vi "ScriptHelper.vi"(11 "Tag":string) -> ()   [LabVIEW 2018]
uses:
  AvailableModules.ctl
  NistPluggableModules/TestClass/Test.lvclass
  NistPluggableModules/Visualization/VisualizeBase/VisualizeBase_class/VisualizeBase.lvclass
panel:
  in  "Select Module":T1
  in  "Available Commands":i32(listbox)
  out "Command Information":string
  # "*Drag and drop Available Commands or selectedexample commands into the script editor"
  # "Available Commands"
  # "Command Information"
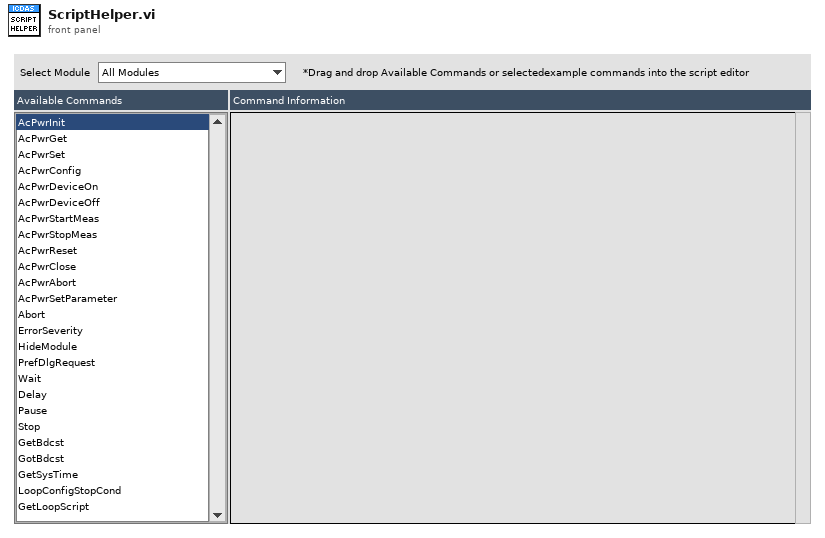
[diagram p1: front panel]
types:
  T1 = typedef "AvailableModules.ctl" = enum16{"All Modules", "AcPwr", "Analysis", "Digitizer", "FGen", "Scope", "Sensor", "Sync"}
  T2 = typedef "Plugin Tree Tag.ctl" = cluster{"ItemType":T3, "Name":string, "Path":path, "Script":string[]}
  T3 = typedef "Plugins Tree Item Type.ctl" = enum16{"Plugin", "Instrument", "INI File", "INI Script"}
  T4 = typedef "Test.lvclass/INIInfo.ctl" = cluster{"Module Name":string, "INI File Name":string, "Class Name":string, "INI File Name Without Extension":string, "Module.Class.INI File Name":string, "Visualization VI Path":path, "Instrument Class Path":path}
  T5 = typedef "Visualization.lvlib/VisualizeBase.lvclass/VisFrmWrkBroadcastEvents.ctl" = cluster{"StatusUpdate":refnum<user-event>, "DidStop":refnum<user-event>, "NewModuleLoaded":refnum<user-event>}
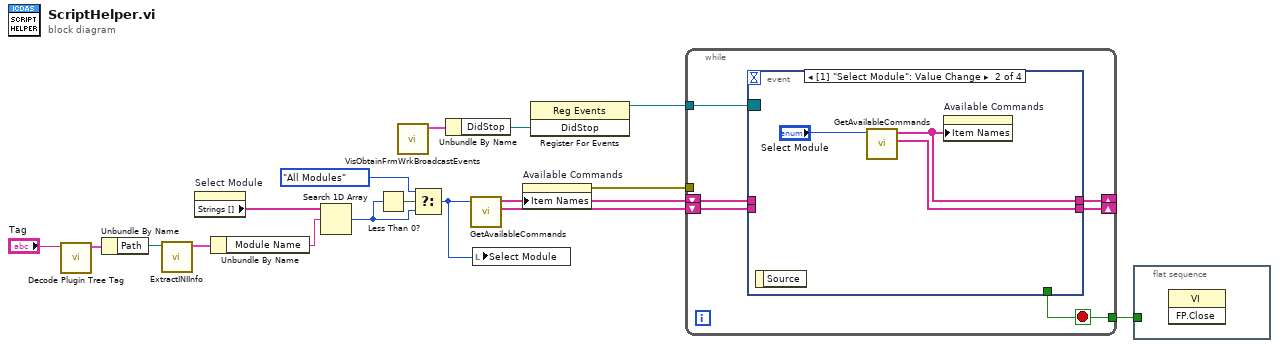
[diagram p0: block diagram]
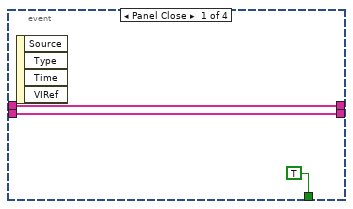
[diagram p2: hidden frame]
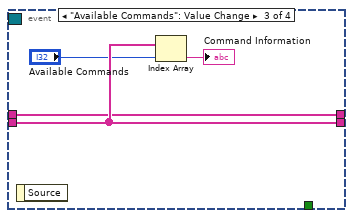
[diagram p3: hidden frame]
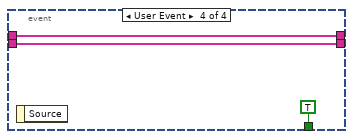
[diagram p4: hidden frame]
diagram:
  n1 = call "Decode Plugin Tree Tag.vi"("Tag"="Tag") -> ("Plugin Tree Tag"=w10:T2)  [unwired: 9 in, 1 out]
  n2 = Unbundle By Name(w10) -> ("Path"=w9:path)
  n3 = call "ExtractINIInfo.vi"("INI File Path"=w9) -> ("INI Info"=w8:T4)  [unwired: 4 in, 6 out]
  n4 = property on="Select Module" class="Enum (strict)"() -> ("Strings []"=w17:string[])  [unwired: 2 in, 2 out]
  n5 = Unbundle By Name(w8) -> ("Module Name"=w1:string)
  n6 = Search 1D Array(1D array=w17, element=w1) -> (index of element=w14:i32)  [unwired: 1 in]
  n7 = Less Than 0?(x=w14) -> (x < 0?=w16:bool)
  n8 = call "VisObtainFrmWrkBroadcastEvents.vi"() -> ("VisFrmWrkBroadcastEvents"=w7:T5)  [unwired: 10 in, 1 out]
  n9 = Select(t=AvailableModules."All Modules" ("Select Module"), s=w16, f=w14) -> (s? t:f=w13:i32)
  n10 = Unbundle By Name(w7) -> ("DidStop"=w6:refnum<user-event>)
  n11 = call "GetAvailableCommands.vi"("Select Module"=w13) -> ("Subdiagram Labels"=w3:string[], "Available Commands"=w2:string[])  [unwired: 9 in]
  n12 = local write "Select Module"(w13) -> ()
  n13 = property on="Available Commands" class="LstBox (strict)"("Item Names"=w2) -> (error out=w12:errorcluster)  [unwired: 2 in, 1 out]
  n14 = register-events(w6) -> (reference out=w5:refnum<event-registration>)  [unwired: 2 in, 1 out]
  n15 = while {
    tunnel: w12 -> [_]
    tunnel: w5 -> [w23]
    tunnel: [w22] -> w4
    shift-right: [w19] -> _
    shift-left: w2 -> [w21]
    shift-right: [w18] -> _
    shift-left: w3 -> [w20]
    stop <- w22 stop-if-true
    n16 = event shown="[1] \"Select Module\": Value Change" {
      selector: w23 -> [_ _ _ _]
      dyn-events: _ -> [_ _ _ _]
      timeout: _ -> [_ _ _ _]
      tunnel: [TRUE _ _ TRUE] -> w22
      tunnel: w21 -> [w25 _ w30 w35]
      tunnel: w20 -> [w24 _ w33 w34]
      tunnel: [w25 w28 w30 w35] -> w19
      tunnel: [w24 w27 w33 w34] -> w18
      event Panel Close {
        n17 = event-data() -> ()  [unwired: 1 in, 4 out]
      }
      event Value Change {
        n18 = event-data() -> ()  [unwired: 1 in, 1 out]
        n19 = call "GetAvailableCommands.vi"("Select Module"="Select Module") -> ("Subdiagram Labels"=w27:string[], "Available Commands"=w28:string[])  [unwired: 9 in]
        n20 = property on="Available Commands" class="LstBox (strict)"("Item Names"=w28) -> ()  [unwired: 2 in, 2 out]
      }
      event "Available Commands": Value Change {
        n21 = event-data() -> ()  [unwired: 1 in, 1 out]
        n22 = Index Array(array=w33, index="Available Commands") -> (element=→"Command Information":string)
      }
      event User Event {
        n23 = event-data() -> ()  [unwired: 1 in, 1 out]
      }
    }
  }
  n24 = flat-sequence {
    tunnel: w4 -> [_]
    frame #0 {
      n25 = invoke class="VI" method="FP.Close"() -> ()  [unwired: 3 in, 3 out]
    }
  }
